vi "Create and Register User Event.vi"(8 "error in":errorcluster, 10 "Payload Data Type":refnum<class "IMessagePayload.lvclass">, 11 "UserEventMessageTransport":refnum<class "UserEventMessageTransport.lvclass">) -> (0 "error out":errorcluster, 3 "UserEventMessageTransport":refnum<class "UserEventMessageTransport.lvclass">)   [LabVIEW 2016, in "UserEventMessageTransport.lvclass"]
uses:
  UserEventMessageTransport.lvclass
  IMessagePayload/IMessagePayload.lvclass
  UserEventMessageTransport.lvclass/UserEventMessageTransport.ctl
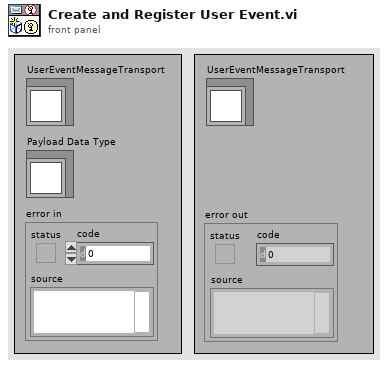
[diagram p1: front panel]
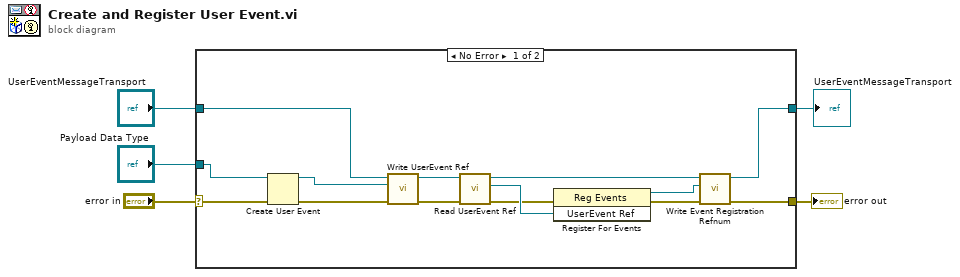
[diagram p0: block diagram]
diagram:
  n1 = case shown="No Error" "error in" {
    selector: "error in" -> [w18 w21]
    tunnel: [w6 w21] -> w4
    tunnel: [w7 w20] -> w2
    tunnel: "UserEventMessageTransport" -> [w16 w20]
    tunnel: "Payload Data Type" -> [w19 _]
    frame No Error {
      n2 = Create User Event(user event datatype=w19, error in=w18) -> (user event=w15:refnum<user-event>, error out=w17:errorcluster)
      n3 = call "Write UserEvent Ref.vi"("error in (no error)"=w17, "UserEvent Ref"=w15, "UserEventMessageTransport"=w16) -> ("error out"=w13:errorcluster, "UserEventMessageTransport"=w14:refnum<class "UserEventMessageTransport.lvclass">)  [unwired: 7 in]
      n4 = call "Read UserEvent Ref.vi"("error in"=w13, "UserEventMessageTransport in"=w14) -> ("error out"=w11:errorcluster, "UserEvent Ref"=w12:refnum<user-event>, "UserEventMessageTransport out"=w8:refnum<class "UserEventMessageTransport.lvclass">)  [unwired: 7 in]
      n5 = register-events(error in=w11, w12) -> (reference out=w9:refnum<event-registration>, error out=w10:errorcluster)  [unwired: 1 in]
      n6 = call "Write Event Registration Refnum.vi"("error in"=w10, "EventRegistration Ref"=w9, "UserEventMessageTransport"=w8) -> ("error out"=w6:errorcluster, "UserEventMessageTransport out"=w7:refnum<class "UserEventMessageTransport.lvclass">)  [unwired: 7 in]
    }
    frame Error {
    }
  }
  "error out" <- w4
  "UserEventMessageTransport" <- w2
